vi "Wait for Trigger.vi"(8 "error in (no error)":errorcluster, 10 "Timeout (10000 ms)":u32=10000, 11 "VISA resource name":refnum<visa-resource-name>) -> (0 "error out":errorcluster, 3 "VISA resource name out":refnum<visa-resource-name>)   [LabVIEW 2018, in "Tektronix TDS 200 1000 2000 Series.lvlib"]
doc: "Waits for the instrument to be triggered only in single acquisition mode. The <B>Timeout</B> control specifies the maximum time to wait for operation complete in milliseconds.\n\n<b>Note(s):</b>\nThis VI will only wait for trigger in single acquisition mode. Does not affect measurements in Continuous acquisition."
uses:
  Tektronix TDS 200 1000 2000 Series.lvlib
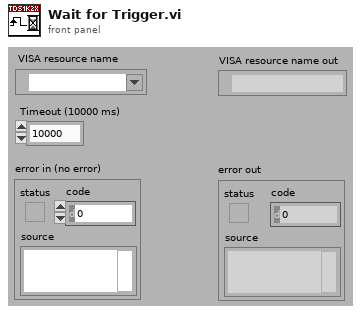
[diagram p1: front panel]
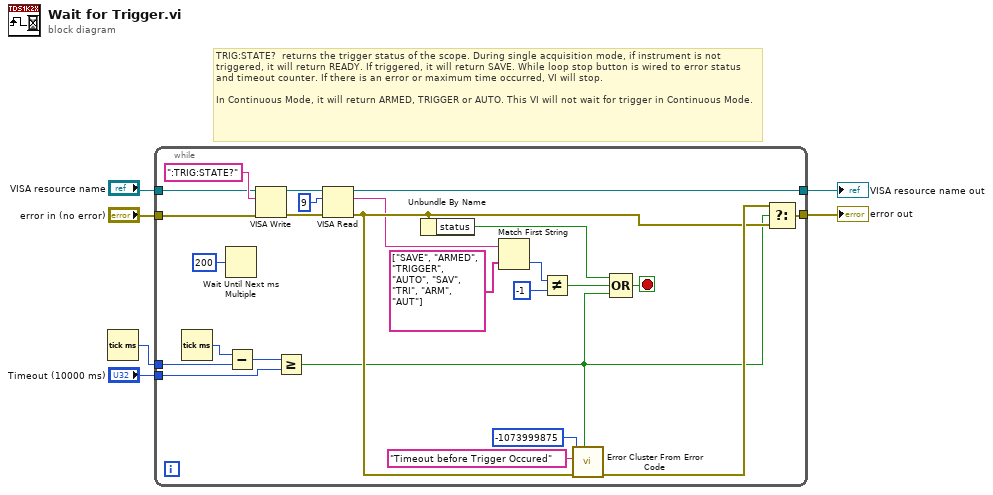
[diagram p0: block diagram]
diagram:
  # "TRIG:STATE?  returns the trigger status of the scope. During single acquisition mode, if instrument is not triggered, it will return READY. If triggered, it will return SAVE. While loop stop button is wired to error status and timeout counter. If there is an error or maximum time occurred, VI will stop.\n\nIn Continuous Mode, it will return ARMED, TRIGGER or AUTO. This VI will not wait for trigger in Continuous Mode."
  n1 = Tick Count (ms)() -> (millisecond timer value=w3:u32)
  n2 = while {
    tunnel: "VISA resource name" -> [w14]
    tunnel: "error in (no error)" -> [w13]
    tunnel: [w27] -> w4
    tunnel: w3 -> [w22]
    tunnel: "Timeout (10000 ms)" -> [w20]
    tunnel: [w17] -> w1
    stop <- w25 stop-if-true
    n3 = Tick Count (ms)() -> (millisecond timer value=w23:u32)
    n4 = Wait Until Next ms Multiple(millisecond multiple=u32 200) -> ()  [unwired: 1 out]
    n5 = Subtract(x=w23, y=w22) -> (x-y=w21:u32)
    n6 = VISA Write(VISA resource name=w14, write buffer=":TRIG:STATE?", error in (no error)=w13) -> (VISA resource name out=w29:refnum<visa-resource-name>, error out=w30:errorcluster)  [unwired: 1 out]
    n7 = Greater Or Equal?(x=w21, y=w20) -> (x >= y?=w7:bool)
    n8 = VISA Read(VISA resource name=w29, byte count=u32 9, error in (no error)=w30) -> (VISA resource name out=w27:refnum<visa-resource-name>, read buffer=w12:string, error out=w15:errorcluster)  [unwired: 1 out]
    n9 = Unbundle By Name(w15) -> ("status"=w24:bool)
    n10 = Match First String(2:string[] ["SAVE", "ARMED", "TRIGGER", "AUTO", "SAV", "TRI", "ARM", "AUT"] ("string array"), 3:w12) -> (0:w10:i32)  [unwired: 1 out]
    n11 = Not Equal?(x=w10, y=-1) -> (x != y?=w8:bool)
    n12 = call "Error Cluster From Error Code.vi"("show call chain? (False)"=w7, "error in (no error)"=w15, "error message (\"\")"="Timeout before Trigger Occured" ("error message (\"\")"), "error code (0)"=-1073999875) -> ("error out"=w16:errorcluster)  [unwired: 5 out]
    n13 = Compound Arithmetic op=OR(w24, w8, w7) -> (w25:bool)
    n14 = Select(t=w16, s=w7, f=w15) -> (s? t:f=w17:errorcluster)
  }
  "error out" <- w1
  "VISA resource name out" <- w4
